vi "macro_SimpleMotorFF_Calculate.vi"   [LabVIEW 2019, in "Trajectory_Library.lvlib"]
uses:
  Trajectory_Library.lvlib
types:
  T1 = typedef "Trajectory_Library.lvlib/SIMPLE_MOTOR_FF.ctl" = cluster{"Ks":dbl, "Kv":dbl, "Ka":dbl}
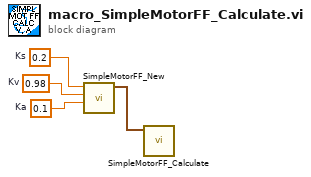
[diagram p0: block diagram]
diagram:
  w1 = 0.2  # Ks
  w2 = 0.98  # Kv
  w3 = 0.1  # Ka
  n1 = call "SimpleMotorFF_New.vi"("Ka"=w3, "Kv"=w2, "Ks"=w1) -> ("SIMPLE_MOTOR_FF"=w4:T1)  [unwired: 8 in]
  n2 = call "SimpleMotorFF_Calculate.vi"("SIMPLE_MOTOR_FF"=w4) -> ()  [unwired: 10 in, 1 out]
